vi "PDLM_GetPulsePowerLimits.vi"(8 "error in (no error)":errorcluster, 11 "USBIdx":i32) -> (0 "error out":errorcluster, 1 "MaxPower":sgl, 2 "MinPower":sgl, 3 "return type":i32)   [LabVIEW 2017]
uses:
  PDLM_DllPath_global.vi
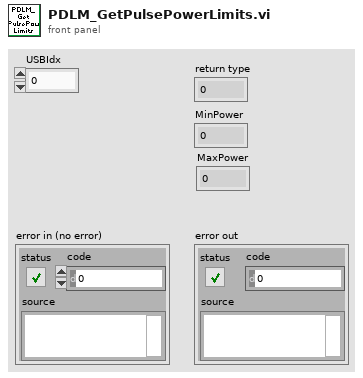
[diagram p1: front panel]
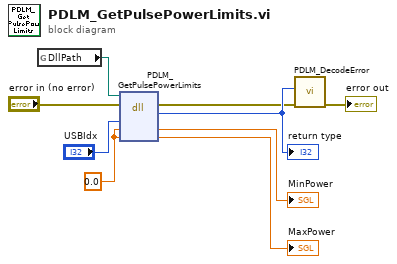
[diagram p0: block diagram]
diagram:
  w1 = sgl 0.0 ("mode")
  n1 = global read "PDLM_DllPath_global.vi" "DllPath"() -> (w5:path)
  n2 = dll-call lib="M:/_dev/progs/LabVIEW/_lib/PQ/Taiko/pdlm_lib.dll" fn="PDLM_GetPulsePowerLimits"(path in=w5, error in="error in (no error)", "USBIdx"="USBIdx", "MinPower"=w1, "MaxPower"=w1) -> (error out=w7:errorcluster, "return type"=w8:i32, "MinPower"=→"MinPower":sgl, "MaxPower"=→"MaxPower":sgl)  [unwired: 2 in, 1 out]
  "return type" <- w8
  n3 = call "PDLM_DecodeError.vi"("error in (no error)"=w7, "code"=w8) -> ("error out"=→"error out":errorcluster)  [unwired: 7 in, 2 out]
